vi "State Machine Example.vi"() -> ()   [LabVIEW 2011]
uses:
  <vilib>/Platform/TimedLoop/XDataNode/timing_clust.ctl
  <vilib>/Platform/TimedLoop/XDataNode/nitl_modes.ctl
  <vilib>/Platform/TimedLoop/XDataNode/wakeup.ctl
  <vilib>/Platform/TimedLoop/XDataNode/XDataNode.xnode
  <vilib>/Platform/TimedLoop/XDataNode/XDNodeRunTimeDep.lvlib
panel:
  out "Input A 2":bool
  out "Input B 2":bool
  out "Enum":enum16{"RESET", "State A"}(ring)
  out "Output A":bool
  out "Output B":bool
  in  "Input A":bool
  in  "Input B":bool
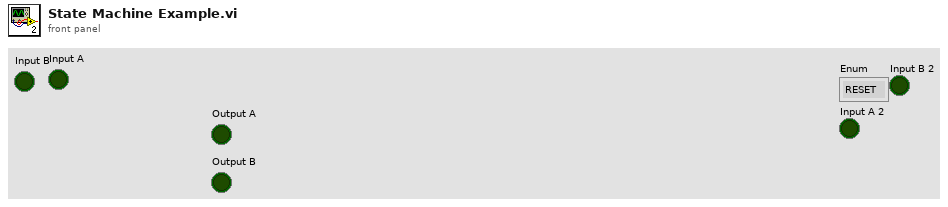
[diagram p1: front panel]
types:
  T1 = typedef "XDNodeRunTimeDep.lvlib/timing_clust.ctl" = cluster{"Expected End [f-1]":u64, "Actual End [f-1]":u64, "Finished Late? [f-1]":bool, "Expected End [i-1]":u64, "Actual End [i-1]":u64, "Finished Late? [i-1]":bool, "Expected Start [i]":u64, "Actual Start [i]":u64, "Expected Start [f]":u64, "Actual Start [f]":u64, "Source Name":string, "Structure Name":string, "Period":i64, "Deadline":i64, "Offset":i64, "Start":i64, "Priority":i32, "Timeout":i32, "Mode":T2, "Wakeup Reason":T3, "Error":errorcluster, "Source Type":string, "Secondary Source Type":string, "Global End Time":u64, "Global Start Time":u64, "Frame Duration":u64, "Iteration Duration":u64, "Assigned CPU":i32, "I/O Scan Engine Mode":u32}
  T2 = typedef "XDNodeRunTimeDep.lvlib/nitl_modes.ctl" = enum32{"No Change", "Process missed periods, maintain original phase", "Discard missed periods, maintain original phase", "Process missed periods, ignore original phase", "Discard missed periods, ignore original phase"}
  T3 = typedef "XDNodeRunTimeDep.lvlib/wakeup.ctl" = enum32{"Normal", "Aborted", "Asynchronous wakeup", "Timing source error", "Timed loop error", "Timeout"}
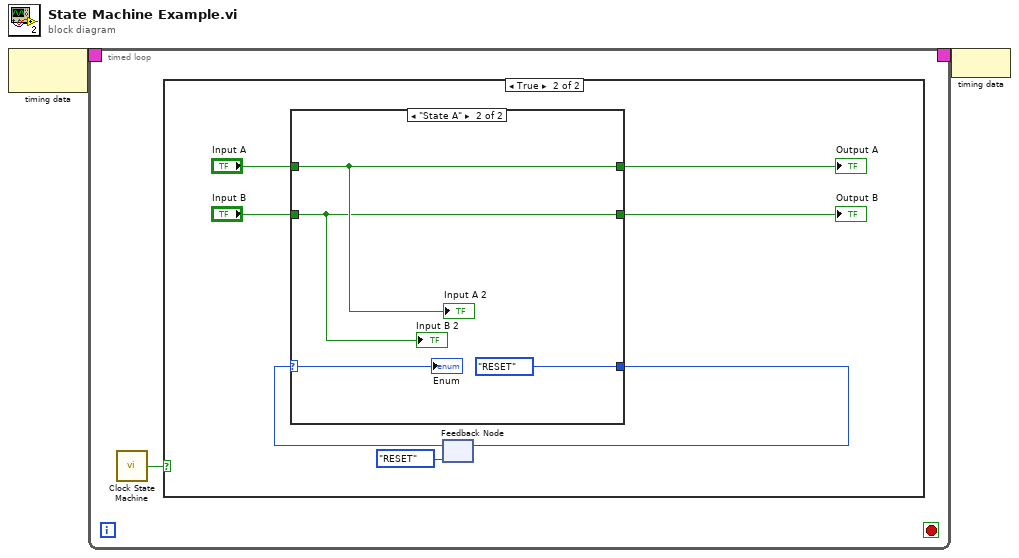
[diagram p0: block diagram]
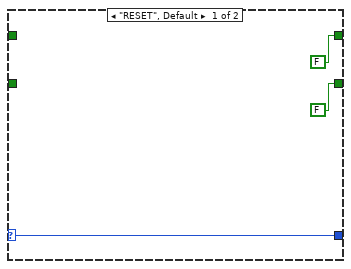
[diagram p3: hidden frame]
diagram:
  n1 = node-c288() -> (w2:T1)  [unwired: 1 in]
  n2 = timed-loop {
    timing: w2 -> [_]
    timing-out: [_] -> w1
    stop <- _ stop-if-true
    n3 = call "Clock State Machine.vi"() -> ("Boolean out"=w3:bool)  [unwired: 15 in]
    n4 = case shown="True" w3 {
      frame False {
      }
      frame True {
        n5 = feedback #1(enum16{"RESET", "State A"}."RESET") -> (w9:enum16{"RESET", "State A"})
        n6 = case shown="\"State A\"" w9 {
          selector: w9 -> [w13 w16]
          tunnel: [w13 enum16{"RESET", "State A"}."RESET"] -> w8
          tunnel: [FALSE ("Input A") w15] -> w7
          tunnel: "Input A" -> [_ w15]
          tunnel: [FALSE ("Input B") w14] -> w5
          tunnel: "Input B" -> [_ w14]
          frame "RESET", Default {
          }
          frame "State A" {
            "Enum" <- w16
            "Input B 2" <- w14
            "Input A 2" <- w15
          }
        }
        "Output A" <- w7
        "Output B" <- w5
        n7 = feedback-in #1(w8) -> ()
      }
    }
  }
  n8 = node-c288(w1) -> ()
